vi "KundtsTube.vi"() -> ()   [LabVIEW 2015]
uses:
  <vilib>/imath/engines/lvmath2/RunTimeEngine/Managers/WorkSpace/UID Generator.vi
  <vilib>/imath/engines/lvmath2/RunTimeEngine/RunTimeType/NIMS_RunTimeType_From StrictType (excl LVString).vi
  <instcachedir>/0/NIMS_RunTimeType_From StrictType (excl LVString)_EB1C38A9BC5048DA9ABDA8F781E54D21.lvgen/NIMS_RunTimeType_From StrictType (excl LVString)_EB1C38A9BC5048DA9ABDA8F781E54D21_000.vi
  <vilib>/imath/engines/lvmath2/RunTimeEngine/LocalVariableDefStatement/MC_LocalVariableDefStatement_Display.vi
  <vilib>/imath/engines/lvmath2/RunTimeEngine/Managers/SymbolTable/Clear UID.vi
  <vilib>/imath/engines/lvmath2/RunTimeEngine/NodeEndStatement/NIMS_NodeEndStatement_Output.vi
  <instcachedir>/0/NIMS_NodeEndStatement_Output_53EC0D466D134D7ABD903AC30B43404B.lvgen/NIMS_NodeEndStatement_Output_53EC0D466D134D7ABD903AC30B43404B_009.vi
  <vilib>/imath/engines/lvmath2/RunTimeEngine/ErrorHandling/NIMS_Finalize Error.vi
  <vilib>/Utility/file.llb/Write Delimited Spreadsheet (DBL).vi
  <vilib>/imath/engines/lvmath2/RunTimeEngine/Managers/SymbolTable/NIMS_WorkSpace.lvlib
panel:
  out "Output Freq":dbl=9930.0
  out "XY Graph":cluster{dbl[], dbl[]}(graph)
  in  "stop":bool
  in  "Amplitude":dbl=5.0
  in  "Pts":dbl=1000.0
  in  "Spacing":u16(ring) items=["Linear", "Logorithmic"]
  in  "Max":dbl=10000.0
  in  "Min":dbl=10.0
  out "RMS":dbl=0.015192168853667603
  out "Waveform Graph":dynamicdata(graph)=[{"t0"=timestamp(3530059620.462291 s since 1904-01-01), "dt"=9.999999999999972e-06, "Y"=array[100000 elements], "attributes"=variant("NI_ChannelName"=variant(string "Voltage"), "NI_UnitDescription"=variant(string "Volts"))}]
  in  "# of Samples":dbl=100000.0
  in  "Sampling Rate":dbl=100000.0
  in  "Tab Control":enum32{"Sweep ", "Single"}(tab)
  in  "Dwell Time Seconds":dbl=0.1
  in  "Frequency":dbl=50.0
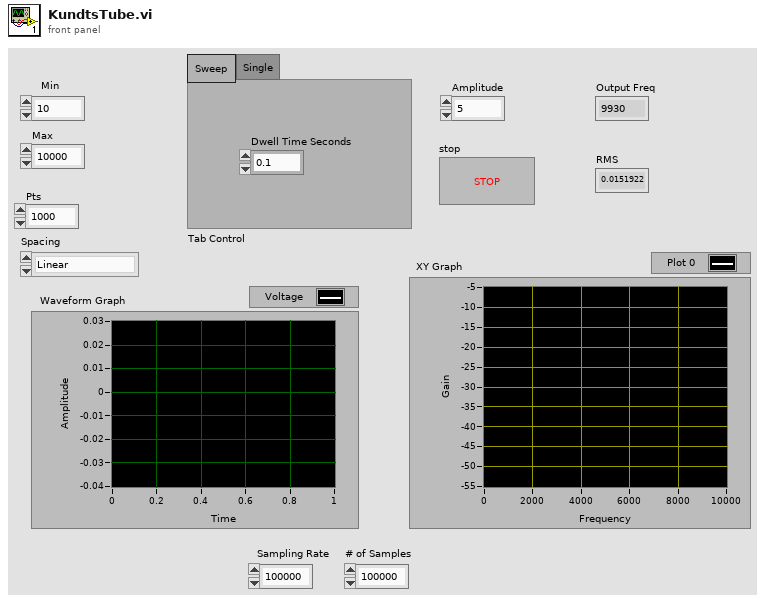
[diagram p1: front panel]
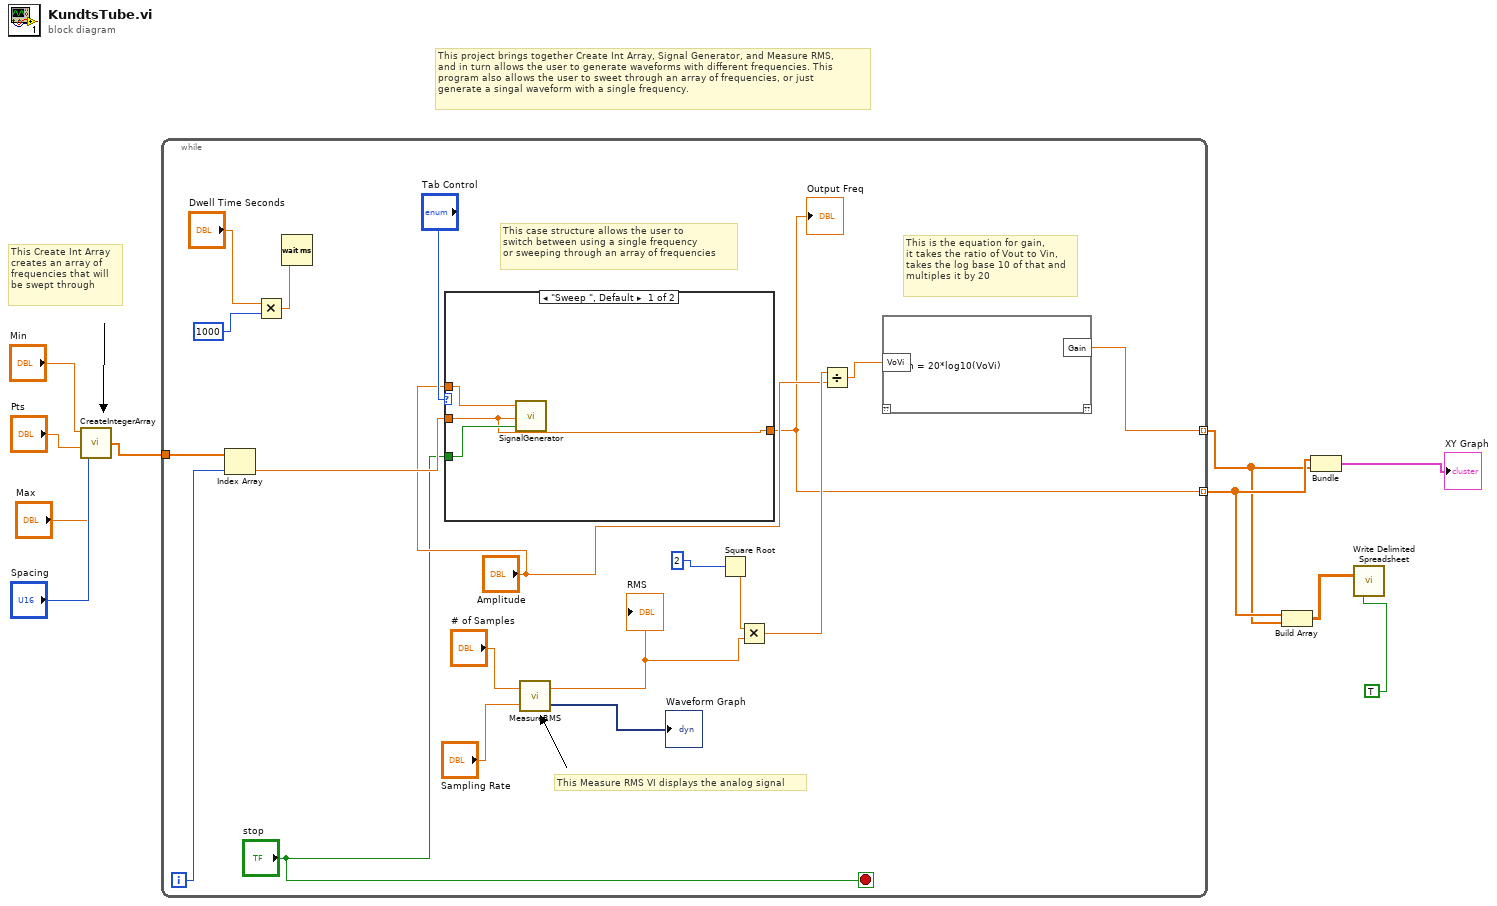
[diagram p0: block diagram]
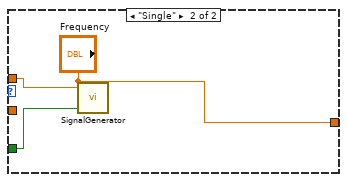
[diagram p2: hidden frame]
diagram:
  # "This Create Int Array \ncreates an array of \nfrequencies that will\nbe swept through"
  # "This project brings together Create Int Array, Signal Generator, and Measure RMS, \nand in turn allows the user to generate waveforms with different frequencies. This\nprogram also allows the user to sweet through an array of frequencies, or just \ngenerate a singal waveform with a single frequency."
  n1 = call "CreateIntegerArray.vi"("Spacing"="Spacing", "Pts"="Pts", "Max"="Max", "Min"="Min") -> ("OutputArray"=w6:dbl[])
  n2 = while {
    tunnel: w6 -> [w25]
    tunnel: [w13] -> w3 mode=indexing
    tunnel: [w12] -> w4 mode=indexing
    i -> [w24]
    stop <- "stop" stop-if-true
    # "This Measure RMS VI displays the analog signal"
    # "This case structure allows the user to\nswitch between using a single frequency \nor sweeping through an array of frequencies"
    # "This is the equation for gain,\nit takes the ratio of Vout to Vin,\ntakes the log base 10 of that and\nmultiples it by 20"
    n3 = Index Array(array=w25, index=w24) -> (element=w23:dbl)
    n4 = Multiply(x="Dwell Time Seconds", y=1000) -> (x*y=w20:dbl)
    n5 = Wait (ms)(milliseconds to wait=w20) -> ()  [unwired: 1 out]
    n6 = case shown="\"Sweep \", Default" "Tab Control" {
      tunnel: "Amplitude" -> [w69 w72]
      tunnel: "stop" -> [w68 w70]
      tunnel: w23 -> [w67 _]
      tunnel: [w67 "Frequency"] -> w12
      frame "Sweep ", Default {
        n7 = call "SignalGenerator.vi"("Boolean"=w68, "Frequency"=w67, "Amplitude"=w69) -> ()
      }
      frame "Single" {
        n8 = call "SignalGenerator.vi"("Boolean"=w70, "Frequency"="Frequency", "Amplitude"=w72) -> ()
      }
    }
    "Output Freq" <- w12
    n9 = call "MeasureRMS.vi"("Sampling Rate"="Sampling Rate", "# of Samples"="# of Samples") -> ("Waveform Graph"=→"Waveform Graph":dynamicdata, "RMS"=w19:dbl)
    "RMS" <- w19
    n10 = Square Root(x=2) -> (sqrt(x)=w17:dbl)
    n11 = Multiply(x=w17, y=w19) -> (x*y=w16:dbl)
    n12 = Divide(x=w16, y="Amplitude") -> (x/y=w14:dbl)
    n13 = mathscript code="Gain = 20*log10(VoVi)"("VoVi"=w14) -> ("Gain"=w13:cdb)  [unwired: 1 in, 1 out]
  }
  n14 = Build Array(w4, w3) -> (w2:cdb[][])
  n15 = Bundle(w4, w3) -> (→"XY Graph":cluster{dbl[], cdb[]})  [unwired: 1 in]
  n16 = call-poly <vilib>:"Write Delimited Spreadsheet.vi"("2D data"=w2, "transpose? (F)"=TRUE) -> ()  [unwired: 12 in, 2 out]
